vi "Write Spectrum Analyzer.lvclass.vi"(10 "Spectrum Analyzer.lvclass":refnum<class "Spectrum Analyzer.lvclass">, 11 "Harmonics in":refnum<class "Harmonics.lvclass">) -> (3 "Harmonics out":refnum<class "Harmonics.lvclass">)   [LabVIEW 2020, in "Harmonics.lvclass"]
uses:
  Harmonics.lvclass
  Instruments/Spectrum Analyzer/Spectrum Analyzer.lvclass
  Harmonics.lvclass/Harmonics.ctl
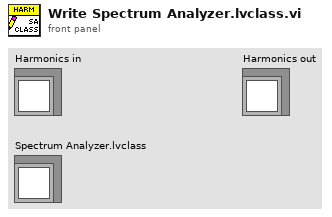
[diagram p1: front panel]
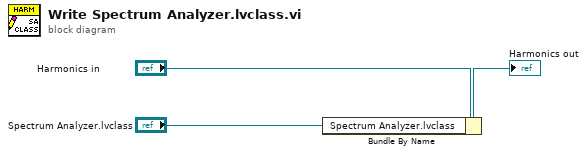
[diagram p0: block diagram]
diagram:
  n1 = Bundle By Name(cluster="Harmonics in", "Spectrum Analyzer.lvclass"="Spectrum Analyzer.lvclass") -> (→"Harmonics out":refnum<class "Harmonics.lvclass">)
